vi "Read Coil.vi"(0 "Refnum in":refnum<visa-resource-name>, 1 "startReg":u16, 2 "Quantity":u16=1, 5 "Mode":T1, 11 "error in (no error)":errorcluster, 12 "Enable":bool) -> (4 "Refnum Out":refnum<visa-resource-name>, 6 "ModeOut":T1, 8 "Coils":bool[](array[boolean]), 15 "error out":errorcluster)   [LabVIEW 2020]
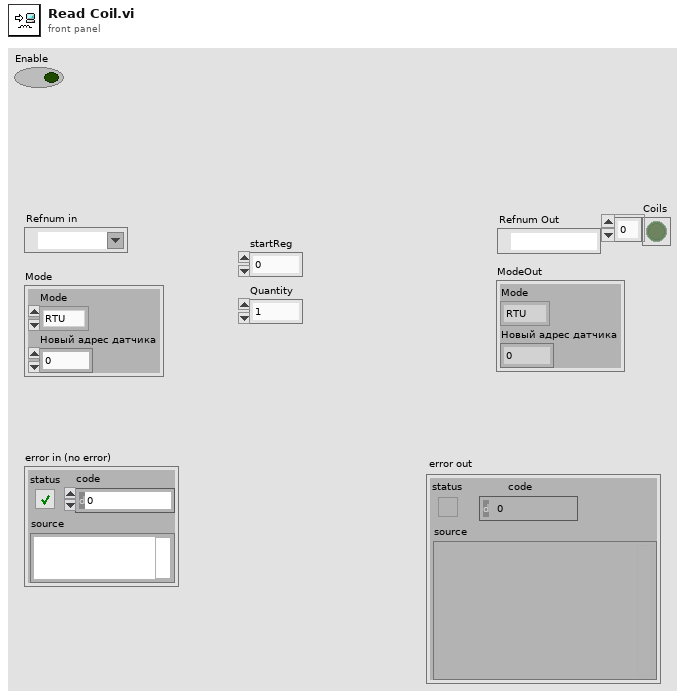
[diagram p1: front panel]
types:
  T1 = cluster{"Mode":enum16{"RTU", "ASCII"}, "Новый адрес датчика":u16}
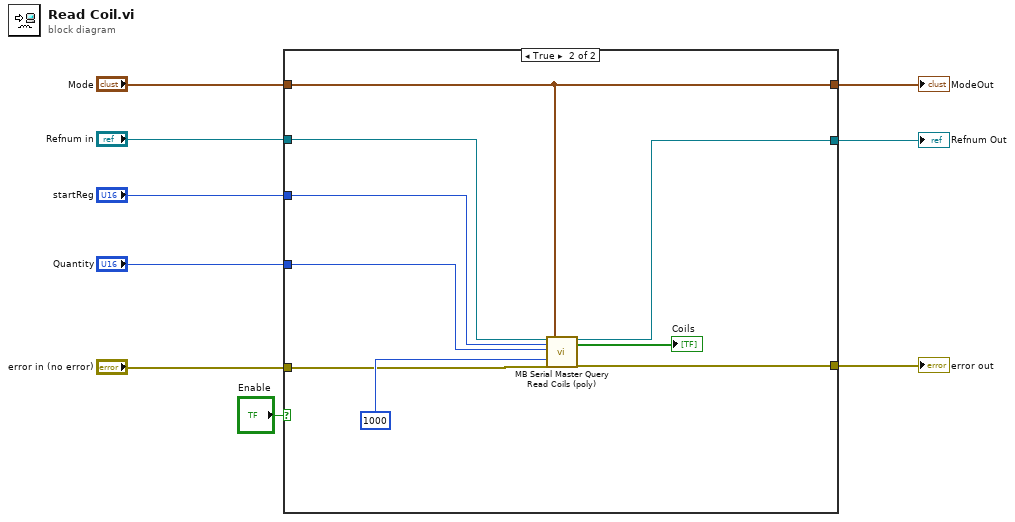
[diagram p0: block diagram]
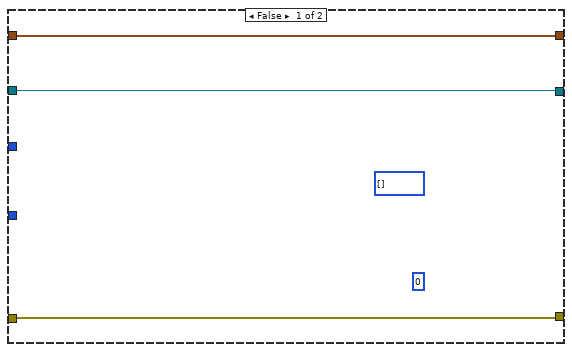
[diagram p2: hidden frame]
diagram:
  n1 = case shown="True" "Enable" {
    tunnel: "Mode" -> [w11 w17]
    tunnel: "error in (no error)" -> [w12 w20]
    tunnel: "Refnum in" -> [w10 w16]
    tunnel: "startReg" -> [_ w19]
    tunnel: "Quantity" -> [_ w14]
    tunnel: [w12 w18] -> w5
    tunnel: [w11 w17] -> w3
    tunnel: [w10 w15] -> w2
    frame False {
      (unwired) u16[] [] ("Holding Registers")
      (unwired) u16 0 ("Numeric")
    }
    frame True {
      n2 = call <vilib>:"MB Serial Master Query Read Coils (poly).vi"("VISA resource name"=w16, "Starting Address"=w19, "Quantity"=w14, "Timeout"=u32 1000, "error in"=w20, "Serial Parameters"=w17) -> ("VISA resource name out"=w15:refnum<visa-resource-name>, "Coils"=→"Coils":bool[], "error out"=w18:errorcluster)  [unwired: 10 in, 1 out]
    }
  }
  "error out" <- w5
  "ModeOut" <- w3
  "Refnum Out" <- w2
